vi "Get Waveform Parameters By Name.vi"(0 "RFSG handle":refnum<k15>, 5 "Waveform Name":string, 11 "error in (no error)":errorcluster) -> (4 "RFSG handle out":refnum<k15>, 6 "Waveform":T1={"Waveform Name"="Wfm", "Waveform"={"x0"=0.0, "dx"=0.0, "y"=[]}, "Signal Bandwidth (Hz)"=0.0, "PAPR (dB)"=0.0, "Burst Length (s)"=0.0, "Sample Rate"=0.0, "Burst Start Locations"=[], "Burst Stop Locations"=[], "Idle Duration Present?"=FALSE, "Runtime Scaling"=0.0} {"Runtime Scaling" format="%#_6p"; "Sample Rate" format="%#_6p"; "Burst Length (s)" format="%#_6p"; "PAPR (dB)" format="%.2f"; "Signal Bandwidth (Hz)" format="%#_6p"; "Waveform"."y" format="%.2f"; "Waveform"."dx" format="%^.2e"; "Waveform"."x0" format="%^.2e"}, 15 "error out":errorcluster)   [LabVIEW 2016, in "SG.lvlib"]
uses:
  SG.lvlib
  Typedefs/Waveform.ctl
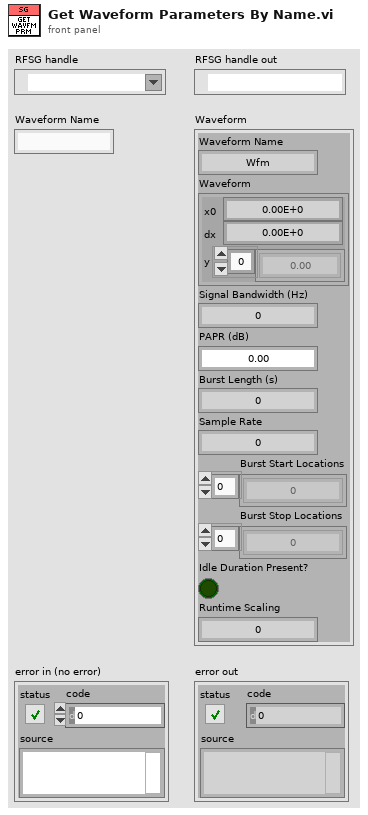
[diagram p1: front panel]
types:
  T1 = typedef "SG.lvlib/Waveform.ctl" = cluster{"Waveform Name":string, "Waveform":cluster{"x0":dbl, "dx":dbl, "y":csg[]}, "Signal Bandwidth (Hz)":dbl, "PAPR (dB)":dbl, "Burst Length (s)":dbl, "Sample Rate":dbl, "Burst Start Locations":i32[], "Burst Stop Locations":i32[], "Idle Duration Present?":bool, "Runtime Scaling":dbl}
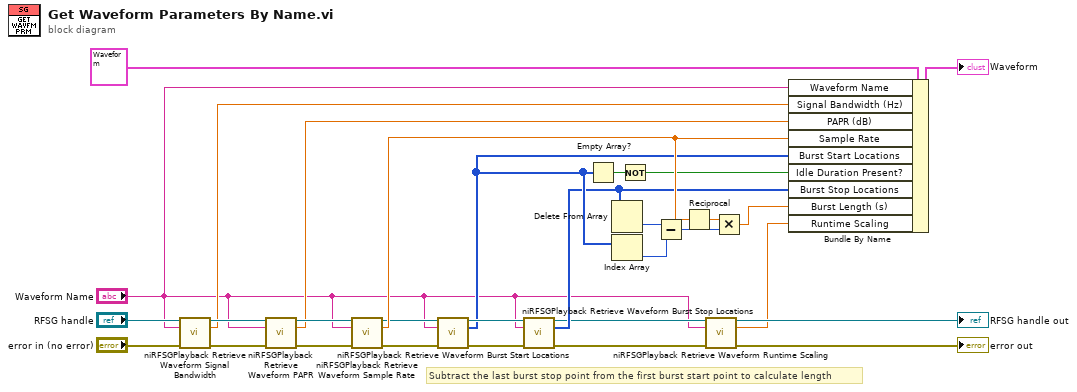
[diagram p0: block diagram]
diagram:
  # "Subtract the last burst stop point from the first burst start point to calculate length"
  n1 = call <instrlib>:"niRFSGPlayback Retrieve Waveform Signal Bandwidth.vi"("instrument handle in"="RFSG handle", "waveform name"="Waveform Name", "error in"="error in (no error)") -> ("instrument handle out"=w27:refnum<k15>, "signal bandwidth"=w17:dbl, "error out"=w23:errorcluster)  [unwired: 10 in]
  n2 = call <instrlib>:"niRFSGPlayback Retrieve Waveform PAPR.vi"("instrument handle in"=w27, "waveform name"="Waveform Name", "error in"=w23) -> ("instrument handle out"=w28:refnum<k15>, "PAPR"=w16:dbl, "error out"=w22:errorcluster)  [unwired: 10 in]
  n3 = call <instrlib>:"niRFSGPlayback Retrieve Waveform Sample Rate.vi"("instrument handle in"=w28, "waveform name"="Waveform Name", "error in"=w22) -> ("instrument handle out"=w26:refnum<k15>, "sample rate"=w30:dbl, "error out"=w21:errorcluster)  [unwired: 10 in]
  n4 = call <instrlib>:"niRFSGPlayback Retrieve Waveform Burst Start Locations.vi"("instrument handle in"=w26, "waveform name"="Waveform Name", "error in"=w21) -> ("instrument handle out"=w25:refnum<k15>, "burst start locations"=w14:i32[], "error out"=w20:errorcluster)  [unwired: 10 in]
  n5 = call <instrlib>:"niRFSGPlayback Retrieve Waveform Burst Stop Locations.vi"("instrument handle in"=w25, "waveform name"="Waveform Name", "error in"=w20) -> ("instrument handle out"=w6:refnum<k15>, "burst stop locations"=w12:i32[], "error out"=w5:errorcluster)  [unwired: 10 in]
  n6 = Empty Array?(array=w14) -> (empty?=w15:bool)
  n7 = Delete From Array(array=w12) -> (deleted portion=w11:i32)  [unwired: 2 in, 1 out]
  n8 = Index Array(array=w14) -> (element=w10:i32)  [unwired: 1 in]
  n9 = Not(x=w15) -> (.not. x?=w13:bool)
  n10 = Subtract(x=w11, y=w10) -> (x-y=w9:i32)
  n11 = Reciprocal(x=w30) -> (1/x=w7:dbl)
  n12 = call <instrlib>:"niRFSGPlayback Retrieve Waveform Runtime Scaling.vi"("instrument handle in"=w6, "waveform name"="Waveform Name", "error in"=w5) -> ("instrument handle out"=→"RFSG handle out":refnum<k15>, "runtime scaling"=w1:dbl, "error out"=→"error out":errorcluster)  [unwired: 10 in]
  n13 = Multiply(x=w7, y=w9) -> (x*y=w8:dbl)
  n14 = Bundle By Name(cluster=T1 {"Waveform Name"="Wfm", "Waveform"={"x0"=0.0, "dx"=0.0, "y"=[]}, "Signal Bandwidth (Hz)"=0.0, "PAPR (dB)"=0.0, "Burst Length (s)"=0.0, "Sample Rate"=0.0, "Burst Start Locations"=[], "Burst Stop Locations"=[], "Idle Duration Present?"=FALSE, "Runtime Scaling"=0.0} ("Waveform"), "Waveform Name"="Waveform Name", "Signal Bandwidth (Hz)"=w17, "PAPR (dB)"=w16, "Sample Rate"=w30, "Burst Start Locations"=w14, "Idle Duration Present?"=w13, "Burst Stop Locations"=w12, "Burst Length (s)"=w8, "Runtime Scaling"=w1) -> (→"Waveform":T1)
